vi "SWAY WRITE FGV.vi"(7 "Enum - Menu":T1, 8 "error in (no error)":errorcluster, 11 "main ref":T2) -> (0 "error out":errorcluster)   [LabVIEW 2025]
uses:
  controls/LAB-IQ UI Data.ctl
  Sway Write enum.ctl
  d526d67c-090a-4194-9932-463c49b325c5.vi
panel:
  out "connection ID":refnum<k16>
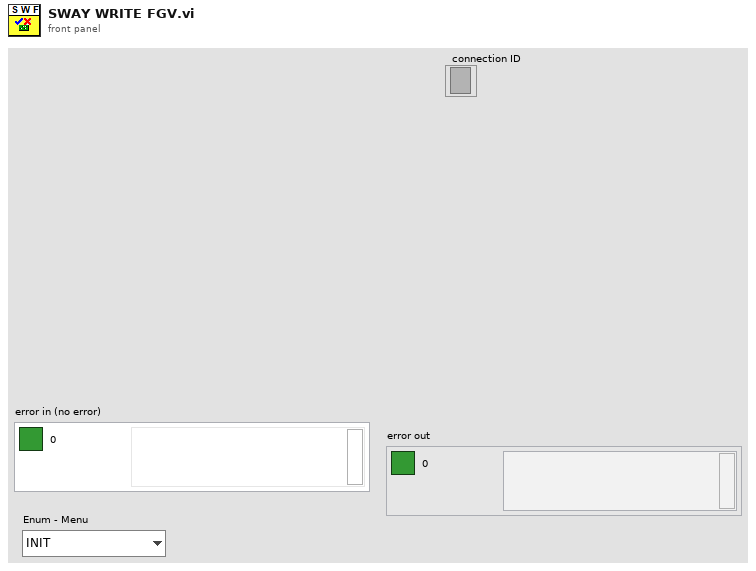
[diagram p1: front panel]
types:
  T1 = typedef "Sway Write enum.ctl" = enum16{"INIT", "READ", "WRITE", "CLOSE", "REINIT"}
  T2 = typedef "LAB-IQ UI Data.ctl" = cluster{"Main Home Screen":cluster{"GUI":refnum<vi>, "Platform Settings":refnum<vi>, "Configure":refnum<vi>, "Home":refnum<vi>, "EXIT":refnum<vi>, "service 2":refnum<vi>, "MainPage":refnum<vi>, "Analysis":refnum<vi>}, "Platform Settings":cluster{"mm/s  Surge":refnum<vi>, "Update Surge Speed":refnum<vi>, "Drive Error":refnum<vi>, "Disable Axis Jog Soft Limits":refnum<vi>, "mm/s  Sway":refnum<vi>, "Sway and Surge COM Status":refnum<vi>, "Heave COM Status":refnum<vi>, "Enable Platform":refnum<vi>, "Surge Forward Main":refnum<vi>, "Sway Right Main":refnum<vi>, "Sway Left Main":refnum<vi>, "Heave Down Main":refnum<vi>, "Heave Up main":refnum<vi>, "Update Sway Speed":refnum<vi>, "Update Heave Speed":refnum<vi>, "mm/s Heave":refnum<vi>, "mm/sec":refnum<vi>, "mm":refnum<vi>, "Surge Backward Main":refnum<vi>}, "Analysis Screen":cluster{"Analysis Home":refnum<vi>, "Surface Analysis":refnum<vi>, "Imaging":refnum<vi>, "Image Analysis":refnum<vi>, "Post Analysis":refnum<vi>}, "Config Screen":cluster{"Select Load Head":refnum<vi>, "Notes :":refnum<vi>, "FILE":refnum<vi>, "Sample ID :":refnum<vi>, "Operator ID :":refnum<vi>, "Operator Name :":refnum<vi>, "Auto":refnum<vi>}, "Motion Module":cluster{"zNL":refnum<vi>, "NL disp":refnum<vi>, "Rotary Tab":refnum<vi>, "Motion Direction:  3":refnum<vi>, "E.Velocity 2":refnum<vi>, "e.v/ssr 2":refnum<vi>, "Enter Fixed E.Velocity 2":refnum<vi>, "Enter Final SRR 2":refnum<vi>, "Enter initial SRR 2":refnum<vi>, "Enter Fixed SRR 2":refnum<vi>, "Enter the Final E.Velocity (m/s) 2":refnum<vi>, "Enter initial E.Velocity (m/s) 2":refnum<vi>, "Final Speed (RPM) 3":refnum<vi>, "Initial Speed (RPM) 2":refnum<vi>, "Enter the Final Velocity (m/s) 3":refnum<vi>, "Enter initial Velocity (m/s)  3":refnum<vi>, "Ramp Up 2":refnum<vi>, "TEST SELECTION":refnum<vi>, "SPEED SELECTION : ":refnum<vi>, "Angular Oscillation Set":refnum<vi>, "Traction":refnum<vi>, "Step Speed":refnum<vi>, "StepTable For Load-Speed":refnum<vi>, "StepTable For Speed":refnum<vi>, "Surge Forward MM":refnum<vi>, "Surge Backward MM":refnum<vi>, "M3 Image":refnum<vi>, "String 39":refnum<vi>, "Sway Left MM":refnum<vi>, "Sway Right MM":refnum<vi>, "Disable Axis Jog Soft Limits":refnum<vi>, "mm":refnum<vi>, "Heave Down MM":refnum<vi>, "Heave Up MM":refnum<vi>, "Wear Track Diameter (mm)":refnum<vi>, "Set WTD":refnum<vi>, "HomeScratch":refnum<vi>, "HomeRot":refnum<vi>, "PlaceModule":refnum<vi>, "Enter the Angle (Deg)":refnum<vi>, "Enter the Frequency (Hz)":refnum<vi>, "Motion Mode:":refnum<vi>, "LR Sway":refnum<vi>, "Rot Hor":refnum<vi>, "Scratch":refnum<vi>, "LR Cam":refnum<vi>, "MMBack":refnum<vi>, "MMNext":refnum<vi>, "Rot Ver":refnum<vi>, "Rotary Module Selection":refnum<vi>, "calculate rotary":refnum<vi>, "SPEED SELECTION : rotary":refnum<vi>, "Import 2":refnum<vi>, "Save 2":refnum<vi>, "File Path :  2":refnum<vi>, "String 45":refnum<vi>, "StepTable For Speed 3":refnum<vi>, "Enter the Speed(mm/sec)":refnum<vi>, "Enter the Speed(RPM)":refnum<vi>, "Enter Scratch Speed (mm/s):":refnum<vi>, "SwaySpeed Set":refnum<vi>, "Scartch Offset":refnum<vi>, "Motion type:":refnum<vi>, "HomeScratch 2":refnum<vi>, "Enter Scratch length (mm):":refnum<vi>, "Wear Track Diameter":refnum<vi>, "Rotary Speed Exced":refnum<vi>, "Scratch Mode":refnum<vi>, "No of Scratch":refnum<vi>}, "Environmental control":cluster{"Humidity  Status  3":refnum<vi>, "Low Temp  Status  2":refnum<vi>, "TK4 status 2":refnum<vi>, "Stage Temperature":refnum<vi>, "Sample Temperature":refnum<vi>, "Humidity (Amb)":refnum<vi>, "Clear List":refnum<vi>, "Add to list":refnum<vi>, "Wear":refnum<vi>, "Vibration":refnum<vi>, "Humidity (Chamber)":refnum<vi>, "Temperature (Chamber)":refnum<vi>, "ECR ":refnum<vi>, "Temperature (Amb)":refnum<vi>, "Microphone":refnum<vi>, "Acoustic Emission 3":refnum<vi>, "SNext":refnum<vi>, "APBack":refnum<vi>, "Enter the Temperature (°C):":refnum<vi>, "Enter the Stage \nTemperature (°C):":refnum<vi>, "Enter the Humidity (%Rh):":refnum<vi>, "Low Temp":refnum<vi>, "High Temp":refnum<vi>, "Humidity":refnum<vi>, "Sensors Picked":refnum<vi>}, "About Screen":cluster{"Password":refnum<vi>, "Home Service":refnum<vi>, "Advanced Setting":refnum<vi>, "About Tab":refnum<vi>, "ECR Port:":refnum<vi>, "Ramp Port:":refnum<vi>, "Installation/Replacement completed":refnum<vi>, "Loahead":refnum<vi>, "Heave and Surge COM Port:":refnum<vi>, "Sway COM Port:":refnum<vi>, "Temp Modbus:":refnum<vi>, "Humidity Port:":refnum<vi>, "Edit Gain Constants":refnum<vi>, "Save Gain Constants":refnum<vi>}, "Main Screen":cluster{"Main Screen Tab":refnum<vi>, "Angle and Frequency":refnum<vi>, "Stroke (mm)":refnum<vi>, "Angle (Deg)":refnum<vi>, "Main Speed Tab":refnum<vi>, "MTM MOTOR DISPLAY":refnum<vi>, "Disc Speed (m/sec)":refnum<vi>, "Ball Speed (m/sec)":refnum<vi>, "Disc Speed (RPM)":refnum<vi>, "Ball Speed (RPM)":refnum<vi>, "SPEED TAB":refnum<vi>, "Speed (m/sec)":refnum<vi>, "Set Speed (m/sec)":refnum<vi>, "Speed (RPM)":refnum<vi>, "Set Speed":refnum<vi>, "Time Tab":refnum<vi>, "Time ( HH:MM:SS ) 2":refnum<vi>, "Test Duration":refnum<vi>, "Test Duration 4":refnum<vi>, "TEST CYCLE":refnum<vi>, "TOTAL CYCLES":refnum<vi>, "Set Load (N)":refnum<vi>, "Temp Tabs":refnum<vi>, "Heater":refnum<vi>, "TK4 status":refnum<vi>, "ChamberTemp":refnum<vi>, "SetTmp":refnum<vi>, "Controller  Status":refnum<vi>, "ChamberTemp 2":refnum<vi>, "SetTmp 2":refnum<vi>, "Controller  Status 2":refnum<vi>, "ChamberTemp 3":refnum<vi>, "SetTmp 3":refnum<vi>, "Cooling":refnum<vi>, "Load Communication":refnum<vi>, "Ambient \nTemperature":refnum<vi>, "HumCOMStatus":refnum<vi>, "Ambient\n Humidity":refnum<vi>, "Freq (Hz)":refnum<vi>, "Load En":refnum<vi>, "NLt":refnum<vi>, "zNL 2":refnum<vi>, "Humidity On":refnum<vi>, "humidity disp":refnum<vi>, "Set Humidity":refnum<vi>, "NL disp 2":refnum<vi>, "Humidity On 2":refnum<vi>, "humidity disp 2":refnum<vi>, "Set Humidity 2":refnum<vi>, "NL disp 3":refnum<vi>, "AppLoadSeq scratch":refnum<vi>, "Stop Scratch":refnum<vi>, "ClrLog":refnum<vi>, "Trip Log":refnum<vi>, "STOP":refnum<vi>, "Start Test":refnum<vi>, "Test status":refnum<vi>, "AR Led":refnum<vi>, "Data":refnum<vi>, "Health":refnum<vi>, "Sway COM Status":refnum<vi>, "Heave COM Status":refnum<vi>, "Grp Tab":refnum<vi>, "Sub Graph":refnum<vi>, "SD (mm)":refnum<vi>, "Siliding distance Reset Graph":refnum<vi>, "SDGp":refnum<vi>, "Humidity Reset Graph":refnum<vi>, "HumrGp":refnum<vi>, "Acoustic Emission (mV)":refnum<vi>, "Aqucostic Reset Graph":refnum<vi>, "gACQUOS":refnum<vi>, "ECR RESET":refnum<vi>, "ECR":refnum<vi>, "Temperature Reset":refnum<vi>, "Acoustic Emission (mV) 2":refnum<vi>, "Aqucostic Reset Graph 2":refnum<vi>, "gACQUOS 2":refnum<vi>, "ECR RESET 2":refnum<vi>, "ECR 2":refnum<vi>, "Temperature Reset 2":refnum<vi>, "Temperature (deg c)":refnum<vi>, "Speed Reset Graph":refnum<vi>, "Speed Tab":refnum<vi>, "MTM DISC  SPEED":refnum<vi>, "MTM BALL SPEED":refnum<vi>, "speed mm/sec":refnum<vi>, "Hymidity":refnum<vi>, "Humidity Disable trip":refnum<vi>, "CoF Trip  2":refnum<vi>, "Depth Trip":refnum<vi>, "Weart Deapth":refnum<vi>, "Depth Reset Graph":refnum<vi>, "Weart":refnum<vi>, "Depthz":refnum<vi>, "Depth (µm)":refnum<vi>, "WearGp":refnum<vi>, "NL Trip 2":refnum<vi>, "Load pid":refnum<vi>, "Load Disable Trip":refnum<vi>, "Load Reset Graph":refnum<vi>, "NL Display 4":refnum<vi>, "Main Chart 3":refnum<vi>, "BACK":refnum<vi>, "Depth Trip 2":refnum<vi>, "COF TRIP ":refnum<vi>, "Friction Force (N)":refnum<vi>, "FF Reset Graph":refnum<vi>, "FF Disable Trip":refnum<vi>, "FF TRIP":refnum<vi>, "COF Disable Trip":refnum<vi>, "COF Reset Graph":refnum<vi>, "Start Test Temp":refnum<vi>, "zFF":refnum<vi>, "Friction Force (N) Graph":refnum<vi>, "Coefficient of Friction":refnum<vi>, "Scratch Start Test":refnum<vi>, "FF Tab":refnum<vi>, "Cyclic Friction Force (N)":refnum<vi>, "CZ FF":refnum<vi>, "Cyclic Friction Force (N) Graph":refnum<vi>, "Cyclic Coefficient of Friction":refnum<vi>, "Cyclic FF TRIP":refnum<vi>, "Cyclic FF Disable Trip":refnum<vi>, "cyclic COF Disable Trip":refnum<vi>, "cyclic COF TRIP":refnum<vi>, "cyclic COF Reset Graph":refnum<vi>, "Cyclic FF Reset Graph":refnum<vi>, "Test Trip":refnum<vi>, "Multi Scratch Pass":refnum<vi>, "Scratch Start Recording":refnum<vi>}, "Loading":cluster{"Indentation":refnum<vi>, "Reference Sample":refnum<vi>, "Load Cell Communication Slide":refnum<vi>, "com 3":refnum<vi>, "com":refnum<vi>, "DecaForce COM Status":refnum<vi>, "Update":refnum<vi>, "Clear 3":refnum<vi>, "seq":refnum<vi>, "Stribeck table":refnum<vi>, "Stribeck Table  For loading":refnum<vi>, "Loading Mode":refnum<vi>, "Enter the Final Load (N)":refnum<vi>, "Enter the CoF Trip":refnum<vi>, "Enter the Friction Force Trip":refnum<vi>, "Enter the Normal load Trip":refnum<vi>, "Enter the Load  (N)":refnum<vi>, "KiloForce":refnum<vi>, "DecaForce ":refnum<vi>, "MicroForce":refnum<vi>, "LHBack":refnum<vi>, "LHNext":refnum<vi>, "Enter the Loading Rate (N/min)":refnum<vi>, "Message":refnum<vi>, "Warning 2":refnum<vi>, "SSP 0.75":refnum<vi>, "SSP 0.5":refnum<vi>, "SSP 0.3":refnum<vi>, "Warning":refnum<vi>, "gui GIF":refnum<vi>, "Communication is established":refnum<vi>, "AppLoad 4":refnum<vi>, "Multipoint":refnum<vi>, "Load Selection":refnum<vi>}, "PID":cluster{"Ramp MulFac":refnum<vi>, "pulses LoadDiffRamp(2..10)":refnum<vi>, "PulseControlRamp(diff<=3N)":refnum<vi>, "SetLoadDeadband(%) Load(0-10N)":refnum<vi>, "PID gains out delay (microForce)":refnum<vi>, "Ramp":refnum<vi>, "Gain 2":refnum<vi>, "pulses LoadDiff(2..10)":refnum<vi>, "pulses LoadDiff(11..50)":refnum<vi>, "PulseControl(diff<=3N)":refnum<vi>, "SetLoadDeadband(%)  2":refnum<vi>, "Dummy Run":refnum<vi>, "Vertical load (N)":refnum<vi>, "AutoTune":refnum<vi>, "Offset 3 ":refnum<vi>, "apply load":refnum<vi>, "Offset  3":refnum<vi>, "apply load 2":refnum<vi>, "Enter ByPass Load":refnum<vi>, "reinit 3":refnum<vi>, "output range delay":refnum<vi>, "PID gains out delay":refnum<vi>, "Bypass Load":refnum<vi>, "pulsesSent":refnum<vi>, "pulses ":refnum<vi>, "actpid":refnum<vi>, "gFF Rot":refnum<vi>, "pulses LoadDiff(21..1000)":refnum<vi>, "Delay":refnum<vi>, "deadband":refnum<vi>}, "Config Parameters":cluster{"Tab Control 3":refnum<vi>, "Tab Control 19":refnum<vi>, "SAMPLES":refnum<vi>, "Re-initilaize":refnum<vi>, "Filter ON/OFF":refnum<vi>, "TracHomeSurgeOffsetCounts 10MM":refnum<vi>, "TracHomeSwayOffsetCounts 10MM":refnum<vi>, "Acoustic Emission:":refnum<vi>, "Apply Filter (FF)":refnum<vi>, "Filter% 2":refnum<vi>, "Apply Filter (Load)":refnum<vi>, "Filter% ":refnum<vi>, "Sway distance (mm)":refnum<vi>, "Surge distance (mm)":refnum<vi>, "DataSavingLoopDelay(ms)":refnum<vi>, "SAVE 2":refnum<vi>, "Enter Distance":refnum<vi>, "Sway Counts:":refnum<vi>, "Distance (mm): 3":refnum<vi>, "Surge Counts:":refnum<vi>, "Distance (mm): 2":refnum<vi>, "Distance (mm):":refnum<vi>, "Heave Counts:":refnum<vi>, "LRMHomeSurgeOffsetCounts":refnum<vi>, "LRMHomeSwayOffsetCounts":refnum<vi>, "TracHomeSurgeOffsetCounts 20MM":refnum<vi>, "TracHomeSwayOffsetCounts 20MM":refnum<vi>, "RotHomeSwayOffsetCounts":refnum<vi>, "RotHomeSurgeOffsetCounts":refnum<vi>, "Heave distance":refnum<vi>, "Zmm":refnum<vi>, "Heave Pulses/mm":refnum<vi>, "Surge Pulses/mm":refnum<vi>, "Sway Pulses/mm":refnum<vi>, "Heave Pitch":refnum<vi>, "Surge Pitch":refnum<vi>, "Sway Pitch":refnum<vi>, "Heave PPR":refnum<vi>, "Surge PPR":refnum<vi>, "Sway PPR":refnum<vi>, "Tab Control 5":refnum<vi>, "Tab Control 14":refnum<vi>, "Tab Control 26":refnum<vi>, "AE":refnum<vi>, "Heave Loop Delay":refnum<vi>, "Heave PID Speed":refnum<vi>, "Surge Jog Speed":refnum<vi>, "Heave Jog Speed":refnum<vi>, "Sway Loop Delay":refnum<vi>, "Sway PID Speed":refnum<vi>, "Sway Jog Speed":refnum<vi>, "DEPTH TRIP VALUE":refnum<vi>, "LOAD TRIP VALUE":refnum<vi>, "DEPTH TRIP   ENABLE":refnum<vi>, "LOAD TRIP  ENABLE":refnum<vi>, "CYCLIC FF TRIP VALUE":refnum<vi>, "FF TRIP VALUE":refnum<vi>, "CYCLIC CoF TRIP VALUE":refnum<vi>, "COF TRIP VALUE":refnum<vi>, "CYCLIC COF TRIP  ENABLE":refnum<vi>, "CYCLIC FF TRIP  ENABLE":refnum<vi>, "FF TRIP  ENABLE":refnum<vi>, "COF TRIP  ENABLE":refnum<vi>}, "Loading Com Port":cluster{"ClearAll":refnum<vi>, "Mz(Nm)":refnum<vi>, "My(Nm)":refnum<vi>, "Mx(Nm)":refnum<vi>, "Save Dwell":refnum<vi>, "Mx ":refnum<vi>, "My ":refnum<vi>, "Mz":refnum<vi>, "Fx(N)":refnum<vi>, "Fy(N)":refnum<vi>, "Fz(N)":refnum<vi>, "ZeroAll":refnum<vi>, "Acq Delay (ms)":refnum<vi>, "Burst Delay (ms)":refnum<vi>, "model":refnum<vi>, "SN":refnum<vi>, "FFx(N)":refnum<vi>, "Sensor IP":refnum<vi>, "Port":refnum<vi>, "FFy(N)":refnum<vi>, "Load(N)":refnum<vi>, "delete Handle":refnum<vi>, "Create Handle":refnum<vi>, "ft_data":refnum<vi>, "ft_range":refnum<vi>, "ft_data 2":refnum<vi>, "stop 6":refnum<vi>, "running_flag":refnum<vi>, "ft_udp_handle":refnum<vi>, "get-data-return":refnum<vi>, "get-range-return":refnum<vi>, "zero-return":refnum<vi>, "filter-return":refnum<vi>, "initial-return":refnum<vi>, "deleteHandle-result":refnum<vi>, "Load Cell Temp":refnum<vi>}, "Heave AND Surge":cluster{"SURGE POSE":refnum<vi>, "error out Read":refnum<vi>, "HEAVE POSE":refnum<vi>, "State":refnum<vi>, "Homed":refnum<vi>, "Sequence ID":refnum<vi>, "error out Write":refnum<vi>, "faultCode":refnum<vi>, "Ack ID":refnum<vi>, "SPEED":refnum<vi>, "Distance":refnum<vi>, "Mode Command":refnum<vi>, "Heave and Surge Read":refnum<vi>, "Read Heave Temp":refnum<vi>, "Spare 15":refnum<vi>, "Spare 14":refnum<vi>, "Spare 13":refnum<vi>, "Spare 12":refnum<vi>, "Spare 11":refnum<vi>, "Spare 10":refnum<vi>, "Spare 9":refnum<vi>, "Spare 8":refnum<vi>, "Spare 7":refnum<vi>, "Spare 6":refnum<vi>, "Spare 5":refnum<vi>, "Spare 4":refnum<vi>, "Spare 2":refnum<vi>, "Spare 1":refnum<vi>, "Node Id":refnum<vi>, "Spare 3":refnum<vi>, "SPARE 4":refnum<vi>, "SPARE 3":refnum<vi>, "SPARE 2":refnum<vi>, "SPARE 1":refnum<vi>, "fwMajor":refnum<vi>, "fwMinor":refnum<vi>, "Manual Write":refnum<vi>, "Heave and Surge Write":refnum<vi>}, "New PID LOGIC":cluster{"Fine Tune Zone":refnum<vi>, "PID SDelay":refnum<vi>, "Max_pos_limit":refnum<vi>, "Min_pos_limit":refnum<vi>, "i_limit":refnum<vi>, "pct_scale":refnum<vi>, "Deadband":refnum<vi>, "Kd":refnum<vi>, "Ki":refnum<vi>, "Kp":refnum<vi>, "Current Position":refnum<vi>, "Set Load":refnum<vi>, "Current Load":refnum<vi>, "Pulse delta":refnum<vi>, "Init Step":refnum<vi>, "Max Step Linit":refnum<vi>}, "SWAY ":cluster{"fwMajor":refnum<vi>, "Homed":refnum<vi>, "Rotary POSE":refnum<vi>, "State":refnum<vi>, "SWAY POSE":refnum<vi>, "Ack ID":refnum<vi>, "faultCode":refnum<vi>, "Node Id":refnum<vi>, "fwMinor":refnum<vi>, "Spare 6":refnum<vi>, "Spare 5":refnum<vi>, "Spare 4":refnum<vi>, "Spare 3":refnum<vi>, "Spare 2":refnum<vi>, "Spare 1":refnum<vi>, "Spare 7":refnum<vi>, "SPARE  5":refnum<vi>, "error out Write  SWAY ":refnum<vi>, "error out Read SWAY ":refnum<vi>, "Manual Write SWAY ":refnum<vi>, "SWAY WRITE":refnum<vi>, "SPARE  4":refnum<vi>, "SPARE  3":refnum<vi>, "SPARE 2":refnum<vi>, "SPARE 1":refnum<vi>, "Spare 15":refnum<vi>, "Spare 14":refnum<vi>, "Spare 13":refnum<vi>, "Spare 12":refnum<vi>, "Spare 11":refnum<vi>, "Spare 9":refnum<vi>, "Spare 8":refnum<vi>, "SPEED":refnum<vi>, "Distance":refnum<vi>, "Mode Command":refnum<vi>, "Sequence ID":refnum<vi>, "SWAY READ":refnum<vi>, "Spare 10":refnum<vi>, "Read SWAY Temp":refnum<vi>}, "Analysis Screen":cluster{"Analysis Home":refnum<vi>, "Refresh 2":refnum<vi>, "MEAN 4":refnum<vi>, "SD 4":refnum<vi>, "VARIANCE 4":refnum<vi>, "MEAN  3":refnum<vi>, "SD  3":refnum<vi>, "VARIANCE  3":refnum<vi>, "MEAN 2":refnum<vi>, "SD  2":refnum<vi>, "VARIANCE 2":refnum<vi>, "MEAN":refnum<vi>, "SD":refnum<vi>, "VARIANCE":refnum<vi>, "File 4 Discription":refnum<vi>, "OPEN 4":refnum<vi>, "File Name 4":refnum<vi>, "OPEN 3":refnum<vi>, "File 3 Discription":refnum<vi>, "File Name 3":refnum<vi>, "Y-AXIS":refnum<vi>, "X-AXIS":refnum<vi>, "XY Graph":refnum<vi>, "File Name 2":refnum<vi>, "File Name 1":refnum<vi>, "OPEN 2":refnum<vi>, "OPEN 1":refnum<vi>, "File 1 Discription ":refnum<vi>, "File 2 Discription":refnum<vi>, "Export":refnum<vi>, "File Format":refnum<vi>}}
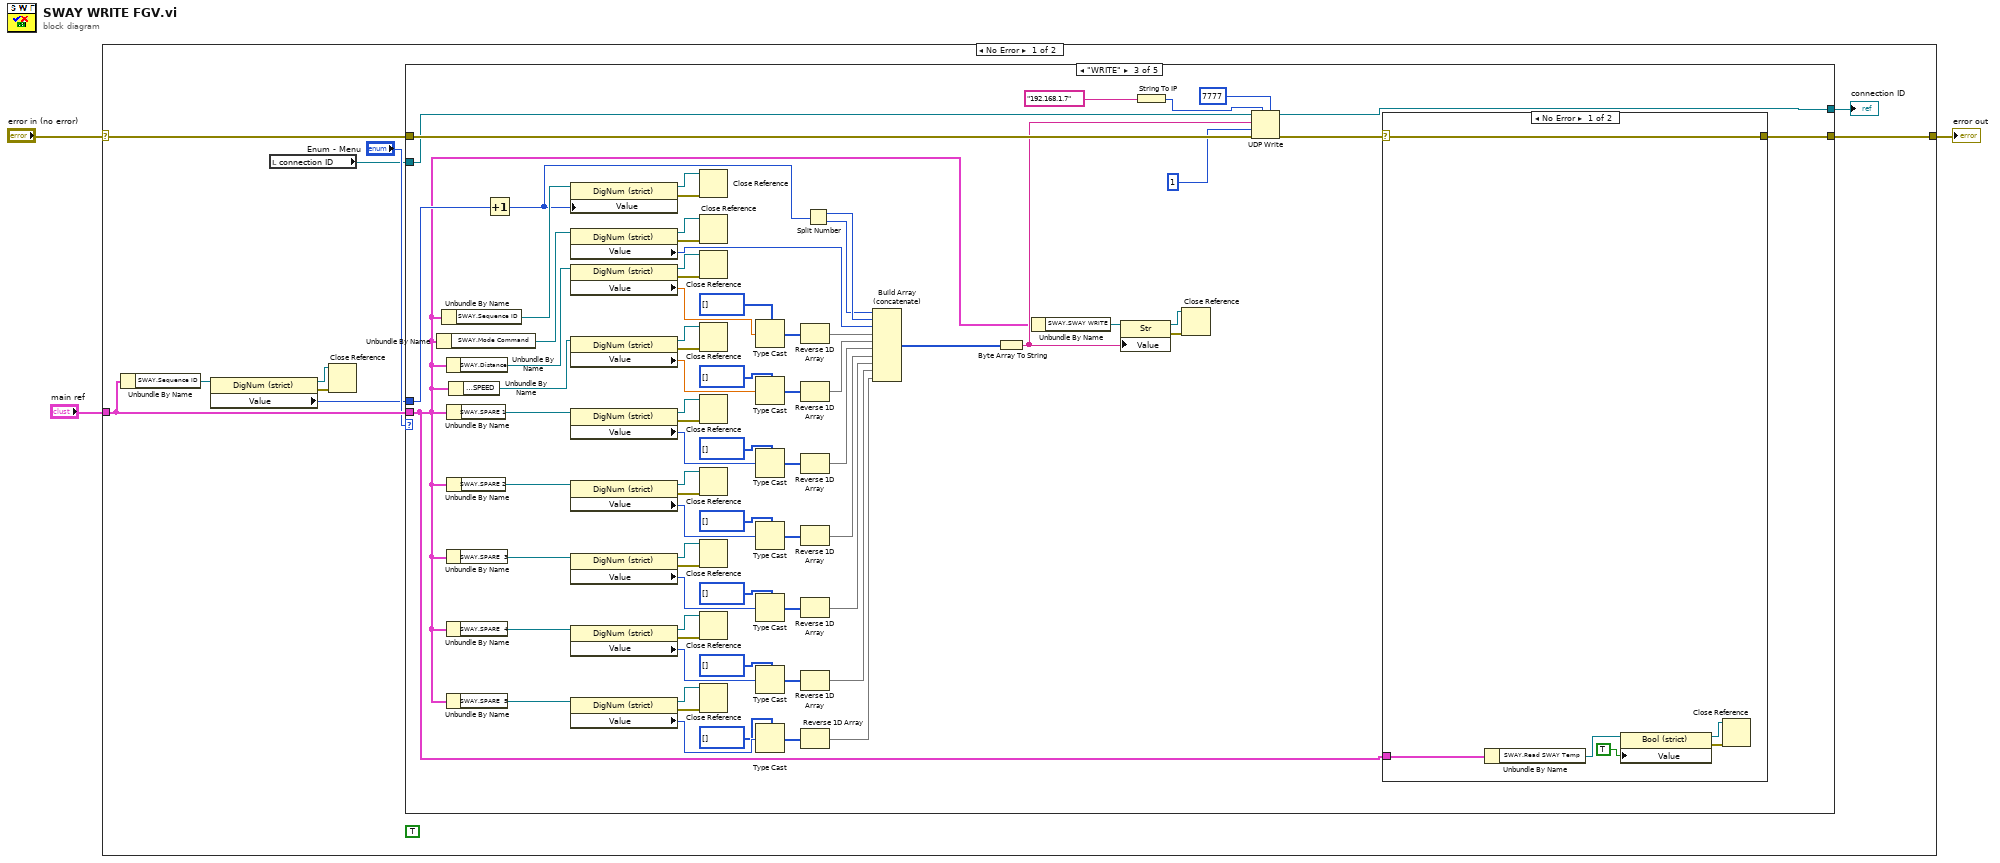
[diagram p0: block diagram]
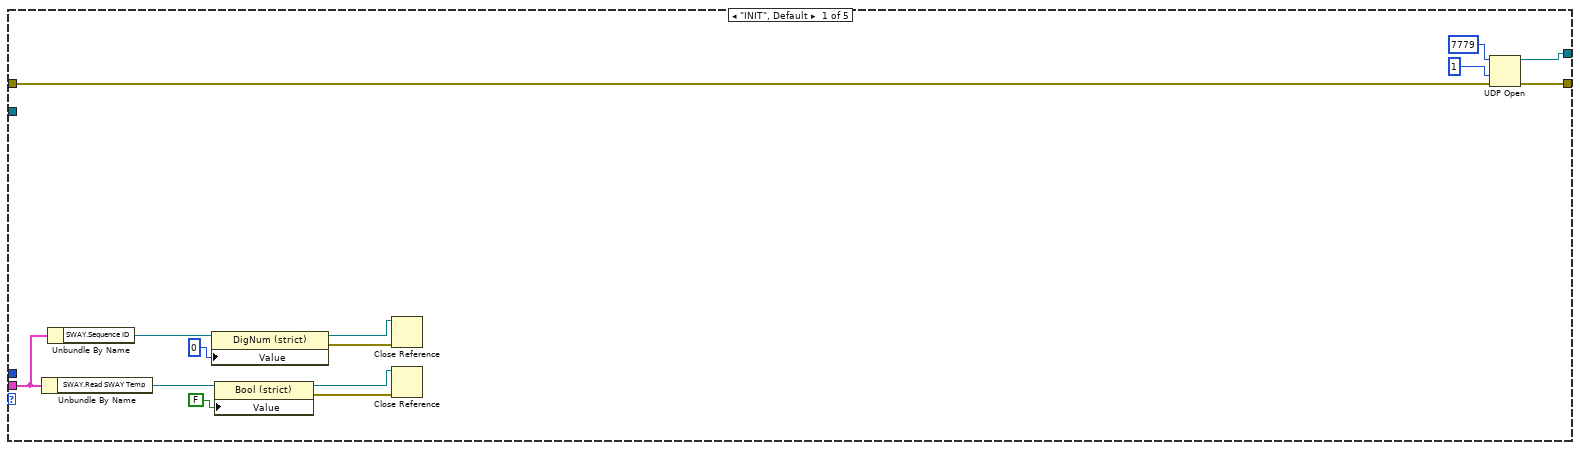
[diagram p2: hidden frame]
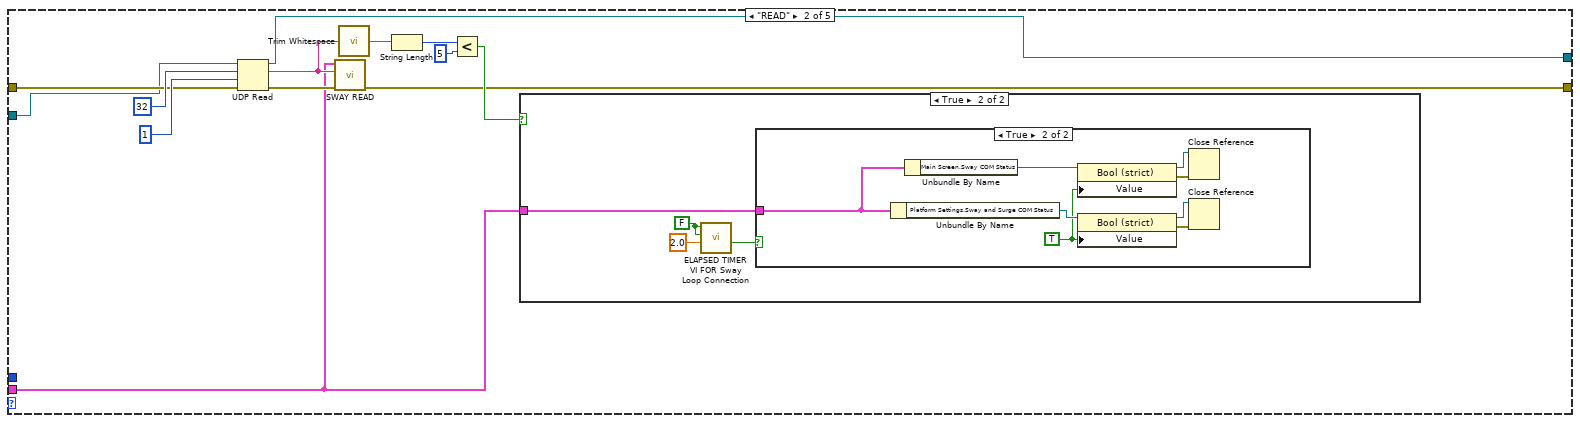
[diagram p3: hidden frame]
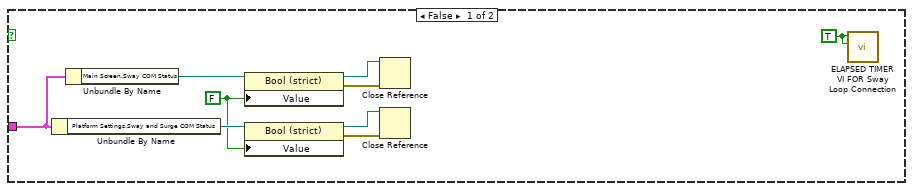
[diagram p4: hidden frame]
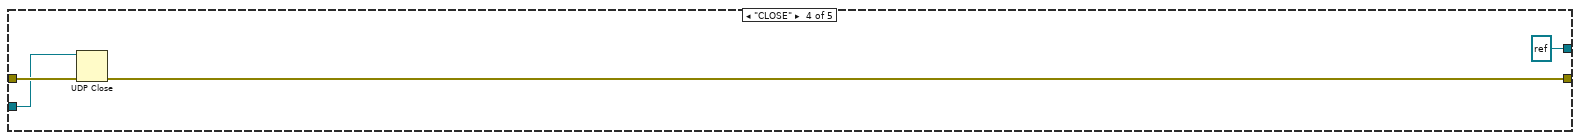
[diagram p7: hidden frame]
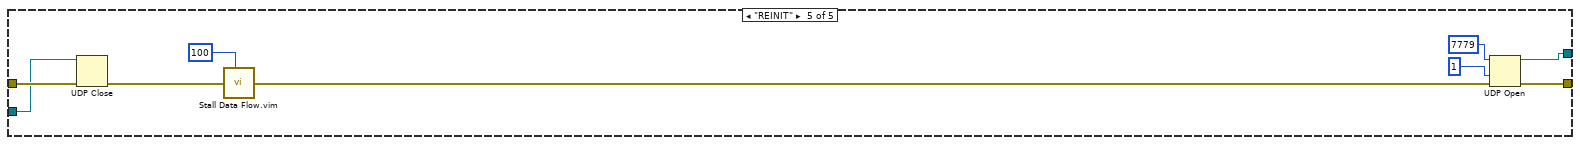
[diagram p8: hidden frame]
diagram:
  n1 = case shown="No Error" "error in (no error)" {
    selector: "error in (no error)" -> [w13 _]
    tunnel: "main ref" -> [w11 _]
    tunnel: [w12 _] -> w1
    frame No Error {
      (unwired) TRUE
      n2 = Unbundle By Name(w11) -> ("SWAY.Sequence ID"=w7:refnum<vi>)
      n3 = property class="DigNum (strict)"(reference=w7) -> (reference out=w9:refnum<vi>, error out=w8:errorcluster, "Value"=w6:u16)  [unwired: 1 in]
      n4 = local read "connection ID"() -> (w5:refnum<k16>)
      n5 = Close Reference(reference=w9, error in (no error)=w8) -> ()  [unwired: 1 out]
      n6 = case shown="\"WRITE\"" "Enum - Menu" {
        tunnel: w13 -> [w26 w32 w134 w146 w155]
        tunnel: [w25 w28 w104 w144 w149] -> w12
        tunnel: [w24 w30 w133 refnum<k16> refnum ("connection ID out") w148] -> w4
        tunnel: w11 -> [w15 w29 w64 _ _]
        tunnel: w6 -> [_ _ w128 _ _]
        tunnel: w5 -> [_ w31 w103 w145 w154]
        frame "INIT", Default {
          n7 = Unbundle By Name(w15) -> ("SWAY.Read SWAY Temp"=w19:refnum<vi>)
          n8 = Unbundle By Name(w15) -> ("SWAY.Sequence ID"=w23:refnum<vi>)
          n9 = property class="DigNum (strict)"(reference=w23, "Value"=u16 0) -> (reference out=w21:refnum<vi>, error out=w22:errorcluster)  [unwired: 1 in]
          n10 = property class="Bool (strict)"(reference=w19, "Value"=FALSE) -> (reference out=w17:refnum<vi>, error out=w18:errorcluster)  [unwired: 1 in]
          n11 = Close Reference(reference=w21, error in (no error)=w22) -> ()  [unwired: 1 out]
          n12 = Close Reference(reference=w17, error in (no error)=w18) -> ()  [unwired: 1 out]
          n13 = UDP Open(8:w26, 9:1 ("timeout ms (25000)"), 11:u16 7779 ("port")) -> (port=w24:refnum<k16>, 0:w25:errorcluster)  [unwired: 2 in, 1 out]
        }
        frame "READ" {
          n14 = UDP Read(connection ID=w31, max size (548)=32, timeout ms (25000)=1, 8:w32) -> (data out=w37:string, error out=w39:errorcluster, 3:w30:refnum<k16>)  [unwired: 2 out]
          n15 = call "SWAY READ.vi"("error in (no error)"=w39, "Heave and Surge Read in"=w37, "Data Cluster"=w29) -> ("error out"=w28:errorcluster)  [unwired: 8 in]
          n16 = call <vilib>:"Trim Whitespace.vi"("string"=w37) -> ("trimmed string"=w38:string)  [unwired: 1 in]
          n17 = String Length(string=w38) -> (length=w36:i32)
          n18 = Less?(x=w36, y=5) -> (x < y?=w34:bool)
          n19 = case shown="True" w34 {
            tunnel: w29 -> [w43 w50]
            frame False {
              w41 = TRUE ("PAUSE")
              w42 = FALSE ("Value")
              n20 = Unbundle By Name(w43) -> ("Platform Settings.Sway and Surge COM Status"=w49:refnum<vi>)
              n21 = Unbundle By Name(w43) -> ("Main Screen.Sway COM Status"=w44:refnum<vi>)
              n22 = property class="Bool (strict)"(reference=w44, "Value"=w42) -> (reference out=w46:refnum<vi>, error out=w45:errorcluster)  [unwired: 1 in]
              n23 = property class="Bool (strict)"(reference=w49, "Value"=w42) -> (reference out=w47:refnum<vi>, error out=w48:errorcluster)  [unwired: 1 in]
              n24 = Close Reference(reference=w46, error in (no error)=w45) -> ()  [unwired: 1 out]
              n25 = Close Reference(reference=w47, error in (no error)=w48) -> ()  [unwired: 1 out]
              n26 = call "ELAPSED TIMER VI FOR Sway Loop Connection.vi"("RESET"=w41, "PAUSE"=w41) -> ()  [unwired: 7 in, 3 out]
            }
            frame True {
              w53 = FALSE ("PAUSE")
              n27 = call "ELAPSED TIMER VI FOR Sway Loop Connection.vi"("TARGET"=2.0, "RESET"=w53, "PAUSE"=w53) -> ("ELAPSED INDICATION"=w51:bool)  [unwired: 6 in, 2 out]
              n28 = case shown="True" w51 {
                tunnel: w50 -> [_ w54]
                frame False {
                }
                frame True {
                  w55 = TRUE ("Value")
                  n29 = Unbundle By Name(w54) -> ("Platform Settings.Sway and Surge COM Status"=w61:refnum<vi>)
                  n30 = Unbundle By Name(w54) -> ("Main Screen.Sway COM Status"=w56:refnum<vi>)
                  n31 = property class="Bool (strict)"(reference=w56, "Value"=w55) -> (reference out=w58:refnum<vi>, error out=w57:errorcluster)  [unwired: 1 in]
                  n32 = property class="Bool (strict)"(reference=w61, "Value"=w55) -> (reference out=w59:refnum<vi>, error out=w60:errorcluster)  [unwired: 1 in]
                  n33 = Close Reference(reference=w58, error in (no error)=w57) -> ()  [unwired: 1 out]
                  n34 = Close Reference(reference=w59, error in (no error)=w60) -> ()  [unwired: 1 out]
                }
              }
            }
          }
        }
        frame "WRITE" {
          n35 = Unbundle By Name(w64) -> ("SWAY.Mode Command"=w123:refnum<vi>)
          n36 = Unbundle By Name(w64) -> ("SWAY.Sequence ID"=w131:refnum<vi>)
          n37 = Unbundle By Name(w64) -> ("SWAY.Distance"=w119:refnum<vi>)
          n38 = Unbundle By Name(w64) -> ("SWAY.SPARE  3"=w93:refnum<vi>)
          n39 = Unbundle By Name(w64) -> ("SWAY.SPARE  4"=w90:refnum<vi>)
          n40 = Unbundle By Name(w64) -> ("SWAY.SPARE  5"=w66:refnum<vi>)
          n41 = Unbundle By Name(w64) -> ("SWAY.SPARE 1"=w99:refnum<vi>)
          n42 = Unbundle By Name(w64) -> ("SWAY.SPARE 2"=w96:refnum<vi>)
          n43 = Unbundle By Name(w64) -> ("SWAY.SPEED"=w112:refnum<vi>)
          n44 = Increment(x=w128) -> (x+1=w127:u16)
          n45 = property class="DigNum (strict)"(reference=w131, "Value"=w127) -> (reference out=w129:refnum<vi>, error out=w130:errorcluster)  [unwired: 1 in]
          n46 = property class="DigNum (strict)"(reference=w123) -> (reference out=w122:refnum<vi>, error out=w124:errorcluster, "Value"=w121:u8)  [unwired: 1 in]
          n47 = property class="DigNum (strict)"(reference=w119) -> (reference out=w120:refnum<vi>, error out=w118:errorcluster, "Value"=w117:sgl)  [unwired: 1 in]
          n48 = property class="DigNum (strict)"(reference=w112) -> (reference out=w113:refnum<vi>, error out=w111:errorcluster, "Value"=w108:sgl)  [unwired: 1 in]
          n49 = property class="DigNum (strict)"(reference=w99) -> (reference out=w98:refnum<vi>, error out=w100:errorcluster, "Value"=w88:u8)  [unwired: 1 in]
          n50 = property class="DigNum (strict)"(reference=w96) -> (reference out=w97:refnum<vi>, error out=w95:errorcluster, "Value"=w85:u8)  [unwired: 1 in]
          n51 = property class="DigNum (strict)"(reference=w93) -> (reference out=w92:refnum<vi>, error out=w94:errorcluster, "Value"=w79:u8)  [unwired: 1 in]
          n52 = property class="DigNum (strict)"(reference=w90) -> (reference out=w91:refnum<vi>, error out=w89:errorcluster, "Value"=w80:u8)  [unwired: 1 in]
          n53 = property class="DigNum (strict)"(reference=w66) -> (reference out=w65:refnum<vi>, error out=w67:errorcluster, "Value"=w70:u8)  [unwired: 1 in]
          n54 = Close Reference(reference=w129, error in (no error)=w130) -> ()  [unwired: 1 out]
          n55 = Close Reference(reference=w122, error in (no error)=w124) -> ()  [unwired: 1 out]
          n56 = Close Reference(reference=w120, error in (no error)=w118) -> ()  [unwired: 1 out]
          n57 = Close Reference(reference=w113, error in (no error)=w111) -> ()  [unwired: 1 out]
          n58 = Close Reference(reference=w98, error in (no error)=w100) -> ()  [unwired: 1 out]
          n59 = Close Reference(reference=w97, error in (no error)=w95) -> ()  [unwired: 1 out]
          n60 = Close Reference(reference=w92, error in (no error)=w94) -> ()  [unwired: 1 out]
          n61 = Close Reference(reference=w91, error in (no error)=w89) -> ()  [unwired: 1 out]
          n62 = Close Reference(reference=w65, error in (no error)=w67) -> ()  [unwired: 1 out]
          n63 = Type Cast(type=u8[] [], x=w117) -> (*(type *) &x=w115:u8[])
          n64 = Type Cast(type=u8[] [], x=w108) -> (*(type *) &x=w110:u8[])
          n65 = Type Cast(type=u8[] [], x=w88) -> (*(type *) &x=w102:u8[])
          n66 = Type Cast(type=u8[] [], x=w85) -> (*(type *) &x=w86:u8[])
          n67 = Type Cast(type=u8[] [], x=w79) -> (*(type *) &x=w81:u8[])
          n68 = Type Cast(type=u8[] [], x=w80) -> (*(type *) &x=w84:u8[])
          n69 = Type Cast(type=u8[] [], x=w70) -> (*(type *) &x=w68:u8[])
          n70 = Reverse 1D Array(array=w115) -> (reversed array=w116:u8[])
          n71 = Reverse 1D Array(array=w110) -> (reversed array=w107:u8[])
          n72 = Reverse 1D Array(array=w102) -> (reversed array=w78:u8[])
          n73 = Reverse 1D Array(array=w86) -> (reversed array=w77:u8[])
          n74 = Reverse 1D Array(array=w81) -> (reversed array=w76:u8[])
          n75 = Reverse 1D Array(array=w84) -> (reversed array=w75:u8[])
          n76 = Reverse 1D Array(array=w68) -> (reversed array=w63:u8[])
          n77 = Split Number(x=w127) -> (hi(x)=w126:u8, lo(x)=w125:u8)
          n78 = Build Array (concatenate)(w125, w126, w121, w116, w107, w78, w77, w76, w75, w63) -> (w106:u8[])
          n79 = Byte Array To String(unsigned byte array=w106) -> (string=w71:string)
          n80 = Unbundle By Name(w64) -> ("SWAY.SWAY WRITE"=w74:refnum<vi>)
          n81 = property class="Str"(reference=w74, "Value"=w71) -> (reference out=w72:refnum<vi>, error out=w73:errorcluster)  [unwired: 1 in]
          n82 = String To IP(1:"192.168.1.7" ("name")) -> (0:w135:u32)
          n83 = Close Reference(reference=w72, error in (no error)=w73) -> ()  [unwired: 1 out]
          n84 = UDP Write(address=w135, port or service name=u16 7777, connection ID=w103, data in=w71, 8:w134, 9:1 ("timeout ms (25000)")) -> (error out=w105:errorcluster, 3:w133:refnum<k16>)
          n85 = case shown="No Error" w105 {
            selector: w105 -> [w142 _]
            tunnel: w64 -> [w137 _]
            tunnel: [w142 _] -> w104
            frame No Error {
              n86 = Unbundle By Name(w137) -> ("SWAY.Read SWAY Temp"=w141:refnum<vi>)
              n87 = property class="Bool (strict)"(reference=w141, "Value"=TRUE) -> (reference out=w139:refnum<vi>, error out=w140:errorcluster)  [unwired: 1 in]
              n88 = Close Reference(reference=w139, error in (no error)=w140) -> ()  [unwired: 1 out]
            }
            frame Error {
            }
          }
        }
        frame "CLOSE" {
          n89 = UDP Close(connection ID=w145, 8:w146) -> (error out=w144:errorcluster)  [unwired: 1 out]
        }
        frame "REINIT" {
          n90 = UDP Close(connection ID=w154, 8:w155) -> (error out=w153:errorcluster)  [unwired: 1 out]
          n91 = call "Stall Data Flow.vim"("value in"=w153, "milliseconds to wait"=u32 100) -> ("value out"=w150:errorcluster)  [unwired: 1 out]
          n92 = UDP Open(8:w150, 9:1 ("timeout ms (25000)"), 11:u16 7779 ("port")) -> (port=w148:refnum<k16>, 0:w149:errorcluster)  [unwired: 2 in, 1 out]
        }
      }
      "connection ID" <- w4
    }
    frame Error {
    }
  }
  "error out" <- w1
